vi "rotation.vi"(7 "On/Off\nRight/Left":bool, 8 "error in (no error)":errorcluster, 11 "angle":ext format="%#_13g") -> (0 "error out":errorcluster, 3 "angle Z":ext)   [LabVIEW 2017]
uses:
  <vilib>/myRIO/Instrument Drivers/Onboard IO/I2C/typedefs/I2C Reference.ctl
  <vilib>/myRIO/Common/Instrument Driver Framework/Utilities/typedefs/myRIO Generic Hardware Reference.ctl
  <vilib>/myRIO/Common/Instrument Driver Framework/Utilities/typedefs/Hardware Version Enum.ctl
  <vilib>/myRIO/Common/Instrument Driver Framework/Utilities/typedefs/myRIO v1.0 Reference.ctl
  <vilib>/myRIO/Common/Instrument Driver Framework/Utilities/typedefs/Generic FPGA Reference.ctl
  <vilib>/myRIO/Common/Instrument Driver Framework/myRIO v1.0/I2C/typedefs/I2C Channels Enum.ctl
  <vilib>/myRIO/Instrument Drivers/Onboard IO/I2C/typedefs/I2C Configuration.ctl
  <vilib>/myRIO/Instrument Drivers/Onboard IO/I2C/typedefs/I2C Transfer Rate.ctl
  <vilib>/userdefined/High Color/nirio_resource_hc.ctl
  <vilib>/myRIO/Common/Instrument Driver Framework/myRIO v1.0/Encoder/typedefs/Encoder Signal Mode.ctl
  <vilib>/myRIO/Instrument Drivers/Onboard IO/Encoder/typedefs/Encoder Reference.ctl
  <vilib>/myRIO/Common/Instrument Driver Framework/myRIO v1.0/Encoder/typedefs/Encoder Channels Enum.ctl
  <vilib>/myRIO/Common/Instrument Driver Framework/myRIO v1.0/Encoder/typedefs/Encoder Configuration v1.0.ctl
  <vilib>/myRIO/Common/Instrument Driver Framework/myRIO v1.0/I2C/vis/myRIO v1.1 Open I2C.vi
  <vilib>/myRIO/Common/Instrument Driver Framework/Utilities/vis/Is FPGA Ref Available.vi
  <vilib>/myRIO/Common/Instrument Driver Framework/myRIO v1.0/Encoder/vis/myRIO v1.1 Open Encoder.vi
  <vilib>/myRIO/Instrument Drivers/Onboard IO/Encoder/vis/Read.vi
  <vilib>/myRIO/Common/Instrument Driver Framework/Utilities/vis/Validate Channels.vi
  <vilib>/myRIO/Common/Instrument Driver Framework/myRIO v1.0/I2C/vis/myRIO v1.0 Reserve I2C.vi
  <vilib>/myRIO/Common/Instrument Driver Framework/myRIO v1.0/Encoder/vis/myRIO v1.0 Reserve Encoder.vi
  <vilib>/myRIO/Common/Instrument Driver Framework/myRIO v1.0/I2C/vis/myRIO v1.0 Close I2C.vi
  <vilib>/myRIO/Common/Instrument Driver Framework/myRIO v1.0/I2C/vis/myRIO v1.0 Build MUX Configuration I2C.vi
  <vilib>/myRIO/Common/Instrument Driver Framework/myRIO v1.0/Resource Manager/vis/myRIO v1.0 Reserve Channel List.vi
  <vilib>/myRIO/Common/Instrument Driver Framework/myRIO v1.0/Encoder/vis/myRIO v1.0 Build MUX Configuration Encoder.vi
  <vilib>/myRIO/Common/Instrument Driver Framework/myRIO v1.0/I2C/vis/myRIO v1.0 Unreserve I2C.vi
  <vilib>/myRIO/Common/Instrument Driver Framework/myRIO v1.0/Resource Manager/vis/myRIO v1.0 Create Configuration List.vi
  <vilib>/myRIO/Common/Instrument Driver Framework/myRIO v1.0/Resource Manager/vis/myRIO v1.0 Reserve Channel.vi
  <vilib>/myRIO/Common/Instrument Driver Framework/myRIO v1.0/Resource Manager/vis/myRIO v1.0 Unreserve Channel.vi
  <vilib>/myRIO/Common/Instrument Driver Framework/myRIO v1.0/Resource Manager/vis/myRIO v1.0 Unreserve Channel List.vi
  <vilib>/myRIO/Common/Instrument Driver Framework/myRIO v1.0/Resource Manager/vis/myRIO v1.0 Build Mutex Name.vi
  <vilib>/Utility/VariantDataType/GetNumericInfo.vi
  <vilib>/Utility/error.llb/Error Cluster From Error Code.vi
  <vilib>/myRIO/Common/Instrument Driver Framework/myRIO v1.0/myRIO v1.1 Open.vi
  <vilib>/myRIO/Common/Instrument Driver Framework/Utilities/vis/IO Manager.vi
  <vilib>/myRIO/Common/Instrument Driver Framework/Utilities/vis/Configuration Manager.vi
  <vilib>/myRIO/Common/Instrument Driver Framework/myRIO v1.0/Resource Manager/vis/myRIO v1.0 Configure IO.vi
  <vilib>/myRIO/Common/Instrument Driver Framework/myRIO v1.0/myRIO v1.0 Close.vi
  <vilib>/myRIO/Common/Instrument Driver Framework/myRIO v1.0/Encoder/vis/myRIO v1.0 Configure Encoder.vi
  <vilib>/myRIO/Common/Instrument Driver Framework/myRIO v1.0/Encoder/vis/myRIO v1.0 Read Encoder.vi
  <vilib>/imath/engines/lvmath2/RunTimeEngine/Managers/WorkSpace/UID Generator.vi
  <vilib>/imath/engines/lvmath2/RunTimeEngine/RunTimeType/NIMS_RunTimeType_From StrictType (excl LVString).vi
  <instcachedir>/0/NIMS_RunTimeType_From StrictType (excl LVString)_1019F277F0A747EDBCA0F6C52CA54500.lvgen/NIMS_RunTimeType_From StrictType (excl LVString)_1019F277F0A747EDBCA0F6C52CA54500_000.vi
  <vilib>/imath/engines/lvmath2/RunTimeEngine/LocalVariableDefStatement/MC_LocalVariableDefStatement_Display.vi
  <vilib>/imath/engines/lvmath2/RunTimeEngine/Managers/SymbolTable/Clear UID.vi
  <vilib>/imath/engines/lvmath2/RunTimeEngine/NodeEndStatement/NIMS_NodeEndStatement_Output.vi
  <instcachedir>/0/NIMS_NodeEndStatement_Output_53EC0D466D134D7ABD903AC30B43404B.lvgen/NIMS_NodeEndStatement_Output_53EC0D466D134D7ABD903AC30B43404B_011.vi
  <vilib>/imath/engines/lvmath2/RunTimeEngine/ErrorHandling/NIMS_Finalize Error.vi
  <vilib>/myRIO/Common/Instrument Driver Framework/myRIO v1.0/I2C/vis/myRIO v1.0 Shutdown I2C.vi
  <vilib>/myRIO/Instrument Drivers/Onboard IO/I2C/vis/myRIO I2C Open.xnode
  <vilib>/myRIO/Express VI/Onboard IO/Encoder/Encoder Express VI.xnode
  <vilib>/myRIO/Instrument Drivers/Onboard IO/Encoder/vis/myRIO Encoder Open.xnode
  <vilib>/myRIO/Common/Instrument Driver Framework/myRIO v1.0/Encoder/typedefs/Encoder Count Direction Enum.ctl
  <vilib>/imath/engines/lvmath2/RunTimeEngine/Managers/SymbolTable/NIMS_WorkSpace.lvlib
  <vilib>/myRIO/Instrument Drivers/Onboard IO/Encoder/Encoder.lvlib
  <vilib>/myRIO/Instrument Drivers/Onboard IO/I2C/I2C.lvlib
panel:
  in  "Stop Motor(false block)":bool
  in  "Stop Motor(true block)":bool
  in  "Stop Button":bool
  out "zMax":ext
  out "zMin":ext
  out "zMin":ext
  out "zMax":ext
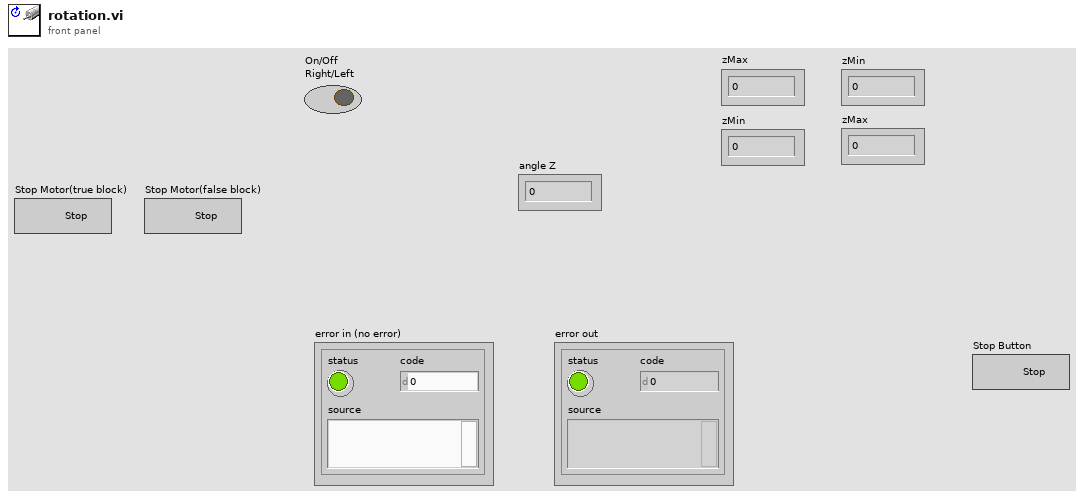
[diagram p1: front panel]
types:
  T1 = typedef "I2C.lvlib/I2C Reference.ctl" = cluster{"myRIO Reference":T2, "I2C Channels Enum":T6, "I2C Configuration":T7}
  T2 = typedef "myRIO Generic Hardware Reference.ctl" = cluster{"myRIO Model":T3, "myRIO Hardware Reference":T4}
  T3 = typedef "Hardware Version Enum.ctl" = enum16{"Unknown", "myRIO-1900", "myRIO-1950", "roboRIO", "NI ELVIS RIO CM"}
  T4 = typedef "myRIO v1.0 Reference.ctl" = cluster{"Generic FPGA Reference":T5, "Allow multiple opens":bool}
  T5 = typedef "Generic FPGA Reference.ctl" = refnum<k20>
  T6 = typedef "I2C Channels Enum.ctl" = enum16{"Not Connected", "A/I2C", "B/I2C", "I2C/I2C"}
  T7 = typedef "I2C.lvlib/I2C Configuration.ctl" = cluster{"I2C Transfer Rate":T8}
  T8 = typedef "I2C.lvlib/I2C Transfer Rate.ctl" = enum16{"Standard mode (100 kbps)", "Fast mode (400 kbps)"}
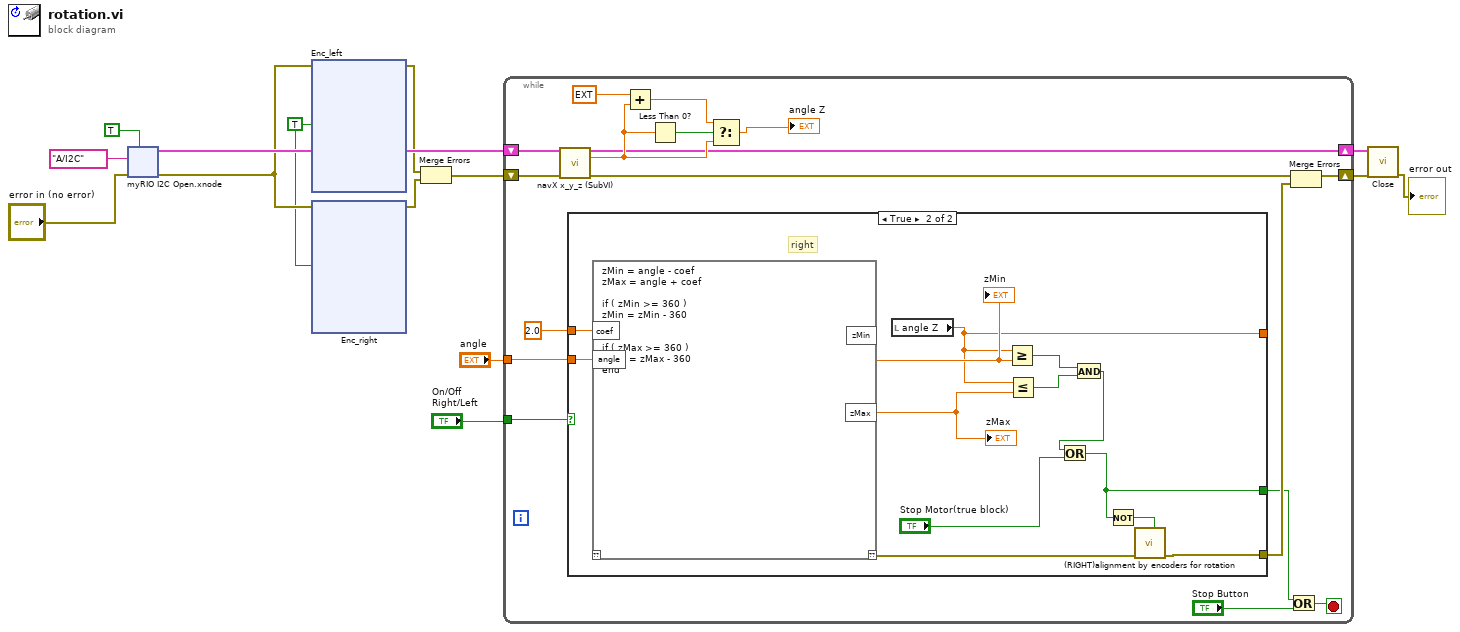
[diagram p0: block diagram]
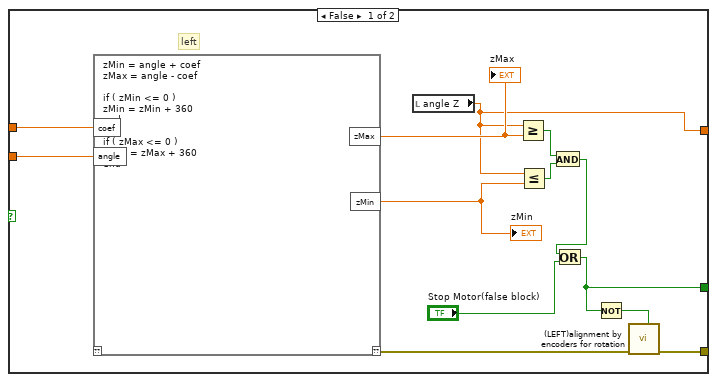
[diagram p2: hidden frame]
diagram:
  w4 = TRUE ("Reset Counter")
  n1 = xnode "myRIO I2C Open.xnode"("error in (no error)"="error in (no error)", "Allow multiple opens?"=TRUE, "Channel Name"=tag "A/I2C") -> ("error out"=w10:errorcluster, "I2C Ref Out"=w12:T1)
  n2 = xnode "Enc_left"("Reset Counter"=w4, "error in (no error)"=w10) -> ("error out"=w5:errorcluster)  [unwired: 3 out]
  n3 = xnode "Enc_right"("Reset Counter"=w4, "error in (no error)"=w10) -> ("error out"=w3:errorcluster)  [unwired: 3 out]
  n4 = Merge Errors(w5, w3) -> (w14:errorcluster)
  n5 = while {
    tunnel: "angle" -> [w25]
    shift-right: [w21] -> w13
    shift-left: w14 -> [w29]
    tunnel: "On/Off\nRight/Left" -> [w20]
    shift-right: [w19] -> w6
    shift-left: w12 -> [w30]
    stop <- w17 stop-if-true
    n6 = call "navX x_y_z (SubVI).vi"("I2C Ref Out in"=w30, "error in (no error)"=w29) -> ("I2C Ref Out out"=w19:T1, "value Z"=w27:ext, "error out"=w22:errorcluster)  [unwired: 9 in, 2 out]
    n7 = case shown="True" w20 {
      tunnel: [w32 w158] -> w15
      tunnel: w25 -> [w44 w168]
      tunnel: 2.0 -> [w41 w167]
      tunnel: [w38 w164] -> _
      tunnel: [w37 w161] -> w23
      frame False {
        # "left"
        n8 = mathscript code="zMin = angle + coef\nzMax = angle - coef\n\nif ( zMin <= 0 )\nzMin = zMin + 360\nend\n\nif ( zMax <= 0 )\nzMax = zMax + 360\nend"("angle"=w44, "coef"=w41) -> ("??"=w36:errorcluster, "zMin"=w39:ext, "zMax"=w40:ext)  [unwired: 1 in]
        "zMin" <- w39
        "zMax" <- w40
        n9 = local read "angle Z"() -> (w38:ext)
        n10 = Greater Or Equal?(x=w38, y=w40) -> (x >= y?=w42:bool)
        n11 = Less Or Equal?(x=w38, y=w39) -> (x <= y?=w43:bool)
        n12 = And(x=w42, y=w43) -> (x .and. y?=w35:bool)
        n13 = Or(x=w35, y="Stop Motor(false block)") -> (x .or. y?=w32:bool)
        n14 = Not(x=w32) -> (.not. x?=w33:bool)
        n15 = call "(LEFT)alignment by encoders for rotation.vi"("On/Off"=w33, "error in (no error)"=w36) -> ("error out"=w37:errorcluster)  [unwired: 9 in]
      }
      frame True {
        # "right"
        n16 = mathscript code="zMin = angle - coef\nzMax = angle + coef\n\nif ( zMin >= 360 )\nzMin = zMin - 360\nend\n\nif ( zMax >= 360 )\nzMax = zMax - 360\nend"("angle"=w168, "coef"=w167) -> ("??"=w160:errorcluster, "zMin"=w165:ext, "zMax"=w166:ext)  [unwired: 1 in]
        "zMax" <- w166
        "zMin" <- w165
        n17 = local read "angle Z"() -> (w164:ext)
        n18 = Greater Or Equal?(x=w164, y=w165) -> (x >= y?=w170:bool)
        n19 = Less Or Equal?(x=w164, y=w166) -> (x <= y?=w169:bool)
        n20 = And(x=w170, y=w169) -> (x .and. y?=w163:bool)
        n21 = Or(x=w163, y="Stop Motor(true block)") -> (x .or. y?=w158:bool)
        n22 = Not(x=w158) -> (.not. x?=w159:bool)
        n23 = call "(RIGHT)alignment by encoders for rotation.vi"("On/Off"=w159, "error in (no error)"=w160) -> ("error out"=w161:errorcluster)  [unwired: 9 in]
      }
    }
    n24 = Add(x=ext 360.0, y=w27) -> (x+y=w26:ext)
    n25 = Less Than 0?(x=w27) -> (x < 0?=w28:bool)
    n26 = Select(t=w26, s=w28, f=w27) -> (s? t:f=→"angle Z":ext)
    n27 = Or(x=w15, y="Stop Button") -> (x .or. y?=w17:bool)
    n28 = Merge Errors(w22, w23) -> (w21:errorcluster)
  }
  n29 = call <vilib>:"Close.vi"("error in (no error)"=w13, "I2C Ref In"=w6) -> ("error out"=→"error out":errorcluster)  [unwired: 9 in]
